vi "SetBoolFeatureValue.vi"(8 "BoolValue":i8, 9 "pFeatureName":string, 10 "handle":i64, 11 "error in (no error)":errorcluster) -> (0 "return type":i32, 3 "error out":errorcluster)   [LabVIEW 2016]
uses:
  MVSDKmd.dll
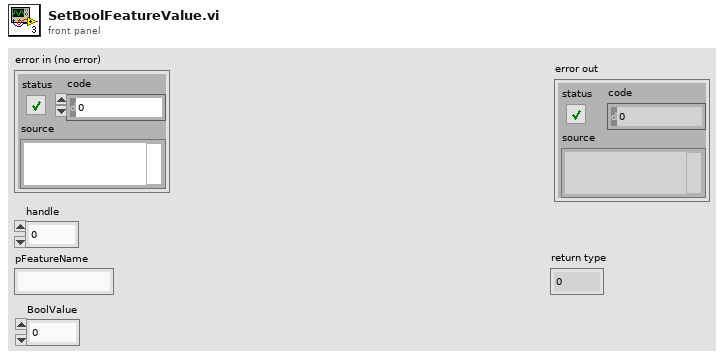
[diagram p1: front panel]
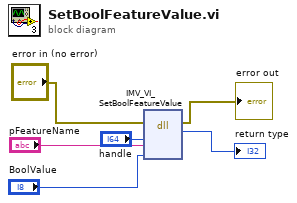
[diagram p0: block diagram]
diagram:
  n1 = dll-call lib="MVSDKmd.dll" fn="IMV_VI_SetBoolFeatureValue"(error in="error in (no error)", "handle"="handle", "pFeatureName"="pFeatureName", "pBoolValue"="BoolValue") -> (error out=→"error out":errorcluster, "return type"=→"return type":i32)  [unwired: 5 in, 1 out]
